vi "Get Server Key File.vi"(11 "gRPC server in":refnum<class "Servicer.lvclass">) -> (2 "Server Key File (.key)":path, 3 "gRPC server out":refnum<class "Servicer.lvclass">)   [LabVIEW 2019, in "gRPC-servicer.lvlib" / "Servicer.lvclass"]
uses:
  Servicer.lvclass
  Servicer.lvclass/Servicer.ctl
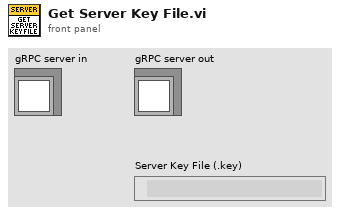
[diagram p1: front panel]
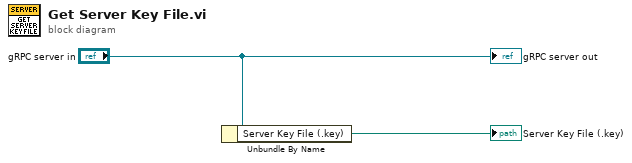
[diagram p0: block diagram]
diagram:
  n1 = Unbundle By Name("gRPC server in") -> ("Server Key File (.key)"=→"Server Key File (.key)":path)
  "gRPC server out" <- "gRPC server in"
